vi "Vision Processing.vi"(4 "error in (no error)":errorcluster, 7 "Image Size":T1=enum."320x240") -> ()   [LabVIEW 2017]
doc: "This VI runs in parallel to other tasks. It gets images from the camera, processes them for color or shape and use that information to affect robot behavior."
uses:
  <vilib>/Rock Robotics/WPI/Camera/WPI_CameraImageSize.ctl
  <vilib>/Rock Robotics/WPI/Camera/WPI_CameraFrameRate.ctl
  <vilib>/Rock Robotics/WPI/Camera/WPI_CameraExposure Values.ctl
  Robot Global Data.vi
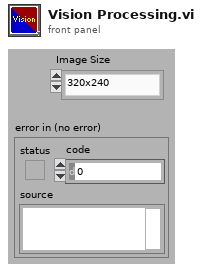
[diagram p1: front panel]
types:
  T1 = typedef "WPI_CameraImageSize.ctl" = enum16{"640x480", "320x240", "160x120", "Custom"}
  T2 = typedef "WPI_CameraExposure Values.ctl" = enum16{"Auto", "Flicker-free 50 Hz", "Flicker-free 60 Hz", "Hold current", "Custom"}
  T3 = typedef "WPI_CameraFrameRate.ctl" = u32
  T4 = typedef "Image Type" = u32
  T5 = typedef "WPI_CameraDevRef.ctl" = cluster{"Camera Address":string, "CameraStatus":errorcluster}
  T6 = typedef "IMAQ Image.ctl" = refnum<image>
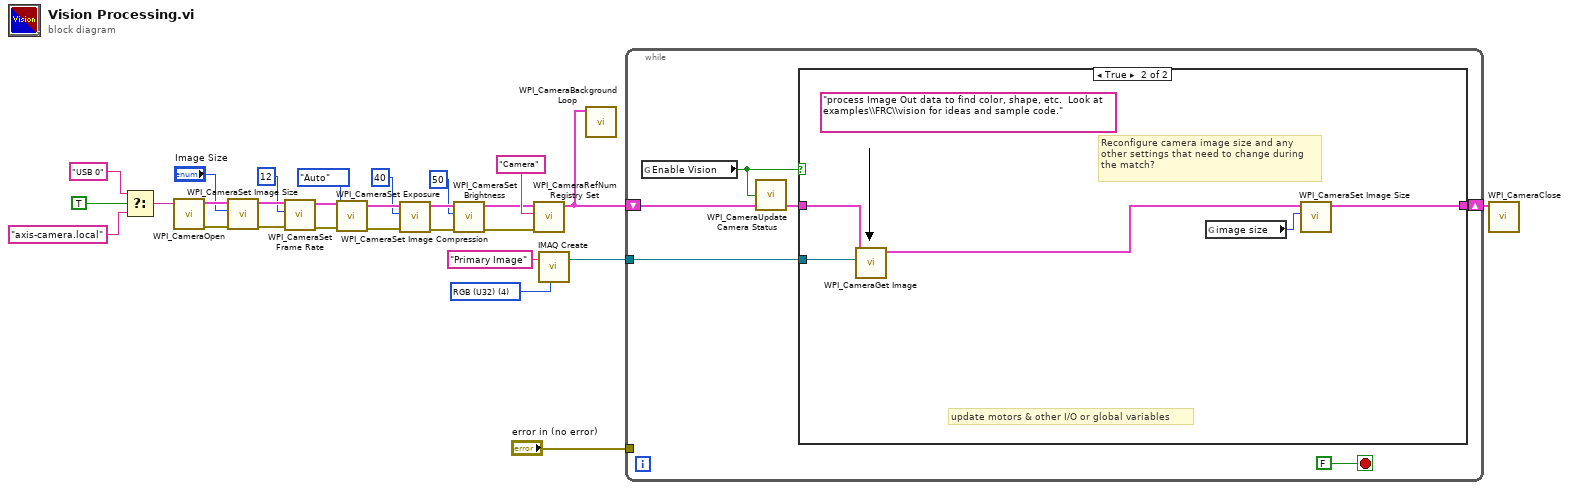
[diagram p0: block diagram]
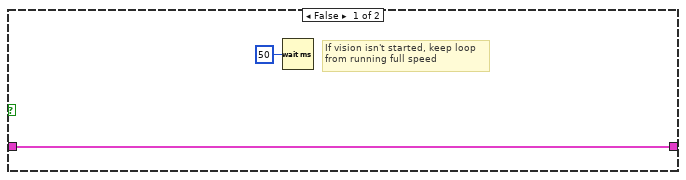
[diagram p2: hidden frame]
diagram:
  w28 = T4 4 items=["Grayscale (U8)", "Grayscale (I16)", "Grayscale (SGL)", "Complex (CSG)", "RGB (U32)", "HSL (U32)", "RGB (U64)"] ("Image Type")
  n1 = Select(t="USB 0" ("format string"), s=TRUE ("dot notation? (F)"), f="axis-camera.local" ("format string")) -> (s? t:f=w16:string)
  n2 = call <vilib>:"WPI_CameraOpen.vi"("Camera Address"=w16) -> ("error out"=w23:errorcluster, "CameraDevRef"=w24:T5)  [unwired: 1 in, 8 out]
  n3 = call <vilib>:"WPI_CameraSet Image Size.vi"("error in (no error)"=w23, "Image Size"="Image Size", "CameraDevRef"=w24) -> ("error out"=w14:errorcluster, "CameraDevRef Out"=w13:T5)  [unwired: 1 in, 6 out]
  n4 = call <vilib>:"WPI_CameraSet Frame Rate.vi"("error in (no error)"=w14, "Frame Rate (fps)"=T3 12, "CameraDevRef"=w13) -> ("error out"=w11:errorcluster, "CameraDevRef Out"=w10:T5)  [unwired: 7 in]
  n5 = call <vilib>:"WPI_CameraSet Exposure.vi"("error in (no error)"=w11, "Exposure"=WPI_CameraExposure_Values."Auto", "CameraDevRef"=w10) -> ("error out"=w7:errorcluster, "CameraDevRef Out"=w8:T5)  [unwired: 7 in]
  n6 = call <vilib>:"WPI_CameraSet Image Compression.vi"("error in (no error)"=w7, "Compression"=40, "CameraDevRef"=w8) -> ("error out"=w5:errorcluster, "CameraDevRef Out"=w4:T5)  [unwired: 7 in]
  n7 = call <vilib>:"WPI_CameraSet Brightness.vi"("error in (no error)"=w5, "Brightness"=50, "CameraDevRef"=w4) -> ("error out"=w1:errorcluster, "CameraDevRef Out"=w2:T5)  [unwired: 7 in]
  n8 = call <vilib>:"WPI_CameraRefNum Registry Set.vi"("error in (no error)"=w1, "refnum name"="Camera", "CameraDevRef"=w2) -> ("CameraDevRef"=w22:T5)  [unwired: 1 in, 7 out]
  n9 = call "IMAQ Create"("Image Name"="Primary Image", "Image Type"=w28) -> ("New Image"=w26:T6)  [unwired: 2 in, 2 out]
  n10 = call <vilib>:"WPI_CameraBackground Loop.vi"("CameraDevRef"=w22) -> ()  [unwired: 11 in]
  n11 = while {
    shift-right: [w33] -> w20
    shift-left: w22 -> [w31]
    tunnel: w26 -> [w32]
    tunnel: "error in (no error)" -> [_]
    stop <- FALSE stop-if-true
    n12 = global read "Robot Global Data.vi" "Enable Vision"() -> (w29:bool)
    n13 = call <vilib>:"WPI_CameraUpdate Camera Status.vi"("CameraDevRef In"=w31, "Enable Vision"=w29) -> ("CameraDevRef Out"=w30:T5)  [unwired: 3 in]
    n14 = case shown="True" w29 {
      tunnel: w32 -> [_ w41]
      tunnel: [w36 w37] -> w33
      tunnel: w30 -> [w36 w39]
      frame False {
        # "If vision isn't started, keep loop\nfrom running full speed"
        n15 = Wait (ms)(milliseconds to wait=u32 50) -> ()  [unwired: 1 out]
      }
      frame True {
        (unwired) "process Image Out data to find color, shape, etc.  Look at examples\\FRC\\vision for ideas and sample code."
        # "update motors & other I/O or global variables"
        # "Reconfigure camera image size and any\nother settings that need to change during\nthe match?"
        n16 = call <vilib>:"WPI_CameraGet Image.vi"("Image"=w41, "CameraDevRef"=w39) -> ("CameraDevRef Out"=w38:T5)  [unwired: 1 in, 8 out]
        n17 = global read "Robot Global Data.vi" "image size"() -> (w40:T1)
        n18 = call <vilib>:"WPI_CameraSet Image Size.vi"("Image Size"=w40, "CameraDevRef"=w38) -> ("CameraDevRef Out"=w37:T5)  [unwired: 2 in, 7 out]
      }
    }
  }
  n19 = call <vilib>:"WPI_CameraClose.vi"("CameraDevRef"=w20) -> ()  [unwired: 1 in, 10 out]
